vi "image_loading.vi"(3 "path to JPEG file":path) -> (1 "image array":T1[](array[typedef]))   [LabVIEW 2018]
uses:
  <vilib>/picture/picture.llb/imagedata.ctl
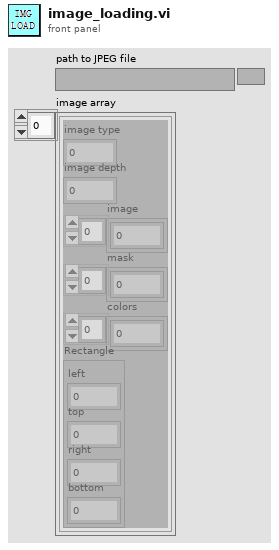
[diagram p1: front panel]
types:
  T1 = typedef "imagedata.ctl" = cluster{"image type":i32, "image depth":i32, "image":u8[], "mask":u8[], "colors":u32[], "Rectangle":cluster{"left":i16, "top":i16, "right":i16, "bottom":i16}}
  T2 = cluster{"left":i16, "top":i16, "right":i16, "bottom":i16}
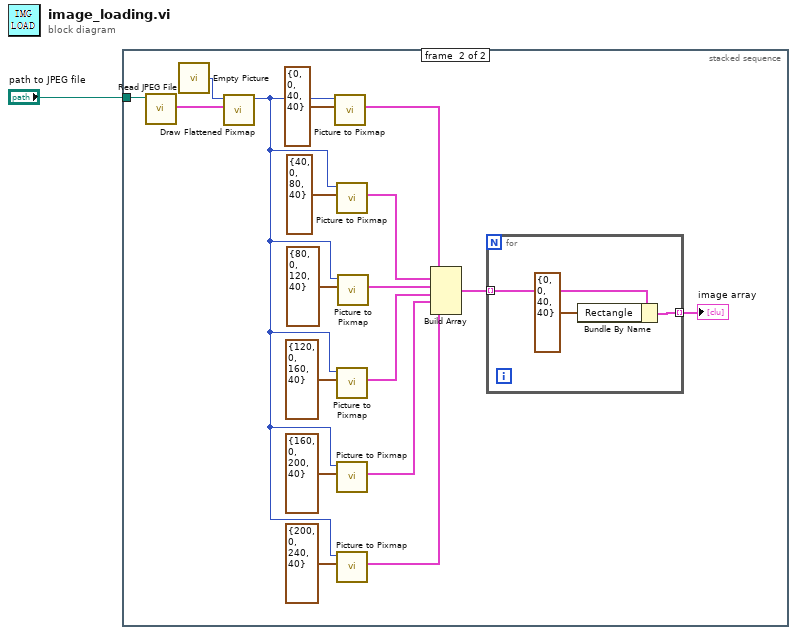
[diagram p0: block diagram]
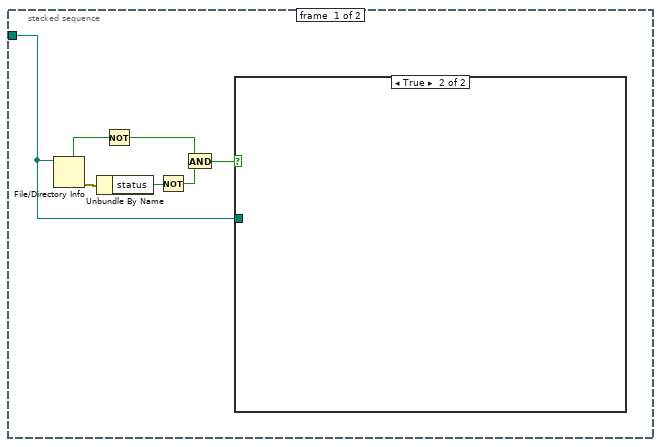
[diagram p2: hidden frame]
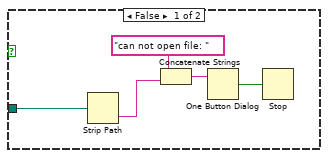
[diagram p3: hidden frame]
diagram:
  n1 = stacked-sequence {
    tunnel: "path to JPEG file" -> [w5 w28]
    frame #0 {
      n2 = File/Directory Info(path=w5) -> (directory=w8:bool, error out=w4:errorcluster)  [unwired: 1 in, 5 out]
      n3 = Unbundle By Name(w4) -> ("status"=w3:bool)
      n4 = Not(x=w8) -> (.not. x?=w7:bool)
      n5 = Not(x=w3) -> (.not. x?=w2:bool)
      n6 = And(x=w7, y=w2) -> (x .and. y?=w6:bool)
      n7 = case shown="True" w6 {
        tunnel: w5 -> [w13 _]
        frame False {
          n8 = Strip Path(path=w13) -> (name=w11:string)  [unwired: 1 out]
          n9 = Concatenate Strings("can not open file: " ("message"), w11) -> (w10:string)
          n10 = One Button Dialog(message=w10) -> (true=w9:bool)  [unwired: 1 in]
          n11 = Stop(stop? (T)=w9) -> ()
        }
        frame True {
        }
      }
    }
    frame #1 {
      n12 = call <vilib>:"Read JPEG File.vi"("path to JPEG file"=w28) -> ("image data"=w31:T1)  [unwired: 8 in, 2 out]
      n13 = call "Empty Picture"() -> ("empty picture"=w30:picture)
      n14 = call <vilib>:"Draw Flattened Pixmap.vi"("image data"=w31, "picture"=w30) -> ("new picture"=w22:picture)  [unwired: 7 in]
      n15 = call <vilib>:"Picture to Pixmap.vi"("rect"=T2 {"left"=0, "top"=0, "right"=40, "bottom"=40}, "picture"=w22) -> ("image data"=w21:T1)  [unwired: 8 in, 1 out]
      n16 = call <vilib>:"Picture to Pixmap.vi"("rect"=T2 {"left"=40, "top"=0, "right"=80, "bottom"=40}, "picture"=w22) -> ("image data"=w20:T1)  [unwired: 8 in, 1 out]
      n17 = call <vilib>:"Picture to Pixmap.vi"("rect"=T2 {"left"=120, "top"=0, "right"=160, "bottom"=40}, "picture"=w22) -> ("image data"=w18:T1)  [unwired: 8 in, 1 out]
      n18 = call <vilib>:"Picture to Pixmap.vi"("rect"=T2 {"left"=160, "top"=0, "right"=200, "bottom"=40}, "picture"=w22) -> ("image data"=w17:T1)  [unwired: 8 in, 1 out]
      n19 = call <vilib>:"Picture to Pixmap.vi"("rect"=T2 {"left"=200, "top"=0, "right"=240, "bottom"=40}, "picture"=w22) -> ("image data"=w16:T1)  [unwired: 8 in, 1 out]
      n20 = call <vilib>:"Picture to Pixmap.vi"("rect"=T2 {"left"=80, "top"=0, "right"=120, "bottom"=40}, "picture"=w22) -> ("image data"=w19:T1)  [unwired: 8 in, 1 out]
      n21 = Build Array(w21, w20, w19, w18, w17, w16) -> (w15:T1[])
      n22 = for {
        tunnel: w15 -> [w34] mode=indexing
        tunnel: [w32] -> w14 mode=indexing
        n23 = Bundle By Name(cluster=w34, "Rectangle"=T2 {"left"=0, "top"=0, "right"=40, "bottom"=40}) -> (w32:T1)
      }
      "image array" <- w14
    }
  }
